vi "process.vi"(8 "error in (no error)":errorcluster, 10 "input":sgl[][](array[numeric]), 11 "DL090628DSSTraceProcessor in":refnum<class "TraceProcessorDL091210Raw.lvclass">) -> (0 "error out":errorcluster, 2 "traces":sgl[][](graph), 3 "DL090628DSSTraceProcessor out":refnum<class "TraceProcessorDL091210Raw.lvclass">)   [LabVIEW 2010, in "TraceProcessorDL091210Raw.lvclass"]
uses:
  TraceProcessorDL091210Raw.lvclass
panel:
  out "current values":sgl[](array[numeric])
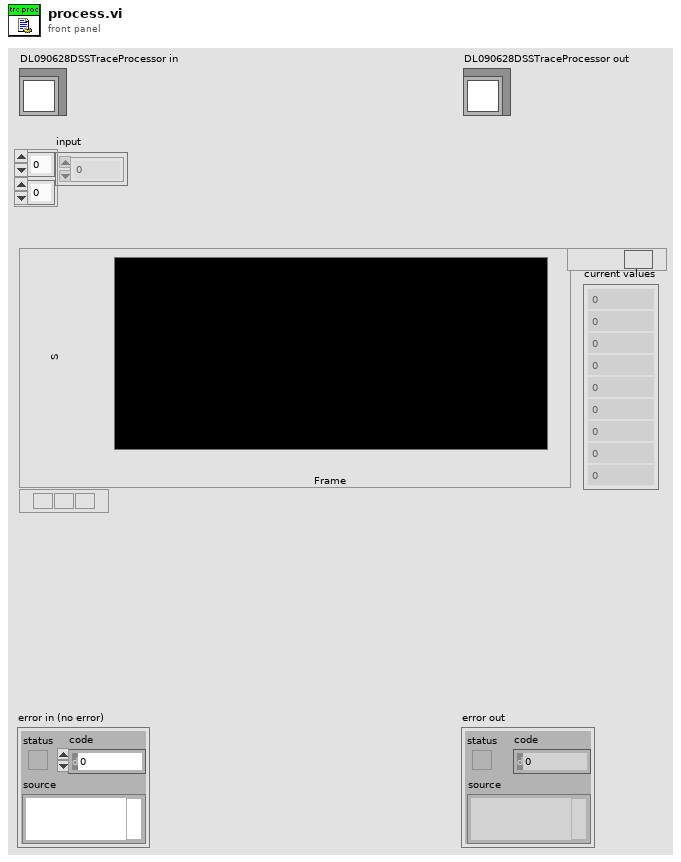
[diagram p1: front panel]
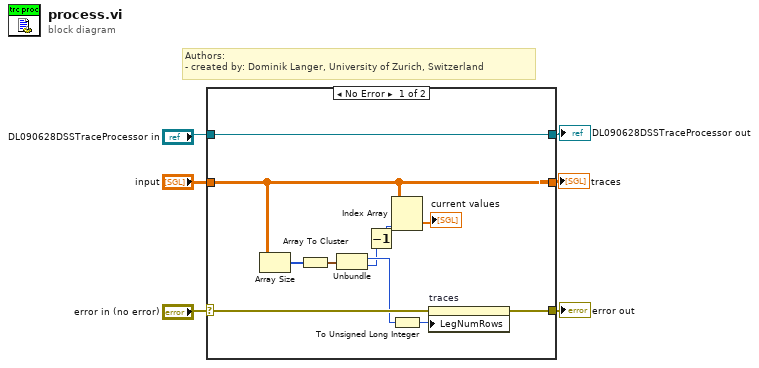
[diagram p0: block diagram]
diagram:
  # "Authors: \n- created by: Dominik Langer, University of Zurich, Switzerland"
  n1 = case shown="No Error" "error in (no error)" {
    selector: "error in (no error)" -> [w16 w19]
    tunnel: [w15 w19] -> w5
    tunnel: [w17 w20] -> w3
    tunnel: "DL090628DSSTraceProcessor in" -> [w17 w20]
    tunnel: "input" -> [w10 w18]
    tunnel: [w10 w18] -> w1
    frame No Error {
      n2 = Array Size(array=w10) -> (size(s)=w13:i32[])
      n3 = Array To Cluster(array=w13) -> (cluster=w12:cluster{"[0]":i32, "[1]":i32})
      n4 = Unbundle(w12) -> ("[0]"=w11:i32, "[1]"=w8:i32)
      n5 = Decrement(x=w8) -> (x-1=w7:i32)
      n6 = Index Array(array=w10, index (col)=w7) -> (element=→"current values":sgl[])  [unwired: 1 in]
      n7 = To Unsigned Long Integer(number=w11) -> (unsigned 32bit integer=w14:u32)
      n8 = property on="traces" class="WFGraph (strict)"(error in=w16, "LegNumRows"=w14) -> (error out=w15:errorcluster)  [unwired: 1 in, 1 out]
    }
    frame Error {
    }
  }
  "error out" <- w5
  "DL090628DSSTraceProcessor out" <- w3
  "traces" <- w1
